vi "Delete LabVIEW Server ID.vi"(7 "Server Alias":string, 10 "Error In":errorcluster) -> (2 "Error Out":errorcluster)   [LabVIEW 2013, in "TS.lvlib"]
uses:
  TS.lvlib
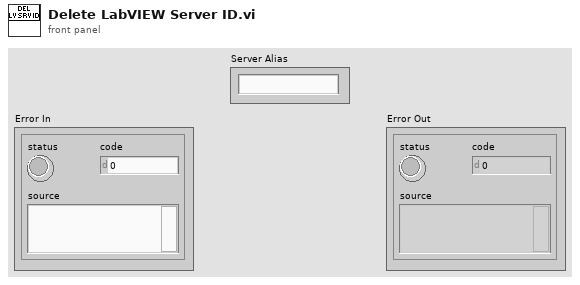
[diagram p1: front panel]
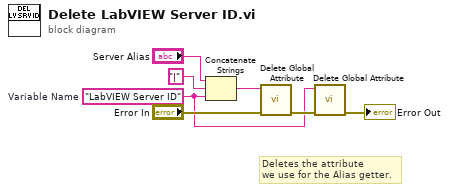
[diagram p0: block diagram]
diagram:
  w2 = "LabVIEW Server ID"  # Variable Name
  # "Deletes the attribute\nwe use for the Alias getter."
  n1 = Concatenate Strings("Server Alias", "|" ("string"), w2) -> (w4:string)
  n2 = call "Delete Global Attribute.vi"("Error In"="Error In", "Name"=w4) -> ("Error Out"=w3:errorcluster)  [unwired: 8 in, 1 out]
  n3 = call "Delete Global Attribute.vi"("Error In"=w3, "Name"=w2) -> ("Error Out"=→"Error Out":errorcluster)  [unwired: 8 in, 1 out]
